vi "Read Data Type Information.vi"(8 "error in (no error)":errorcluster, 10 "Name":string, 11 "TwinCAT ADS in":refnum<class "TwinCAT ADS.lvclass">) -> (0 "error out":errorcluster, 1 "Data Type Information":T1 {"Category" items=["Unknown, None"=0, "Primitive"=1, "Alias"=2, "Enum"=3, "Array"=4, "Struct"=5, "FunctionBlock"=6, "Program"=7, "Function"=8, "SubRange"=9, "String"=10, "Bitset"=12, "Pointer"=13, "Union"=14, "Reference"=15, "Interface"=16]; "Type ID" items=["ADST_VOID"=0, "ADST_INT16"=2, "ADST_INT32"=3, "ADST_REAL32"=4, "ADST_REAL64"=5, "ADST_INT8"=16, "ADST_UINT8"=17, "ADST_UINT16"=18, "ADST_UINT32"=19, "ADST_INT64"=20, "ADST_UINT64"=21, "ADST_STRING"=30, "ADST_WSTRING"=31, "ADST_REAL80"=32, "ADST_BIT"=33, "ADST_MAXTYPES"=34, "ADST_BIGTYPE"=65]}, 3 "TwinCAT ADS out":refnum<class "TwinCAT ADS.lvclass">)   [LabVIEW 2018, in "TwinCAT ADS.lvclass"]
uses:
  TwinCAT ADS.lvclass
  Controls/Data Type Information.ctl
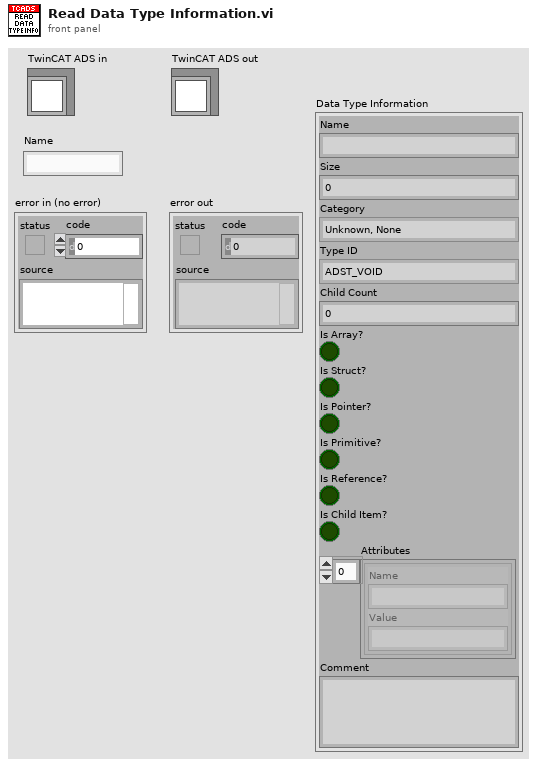
[diagram p1: front panel]
types:
  T1 = typedef "TwinCAT ADS.lvclass/Data Type Information.ctl" = cluster{"Name":string, "Size":i32, "Category":i32, "Type ID":i32, "Child Count":i32, "Is Array?":bool, "Is Struct?":bool, "Is Pointer?":bool, "Is Primitive?":bool, "Is Reference?":bool, "Is Child Item?":bool, "Attributes":cluster{"Name":string, "Value":string}[], "Comment":string}
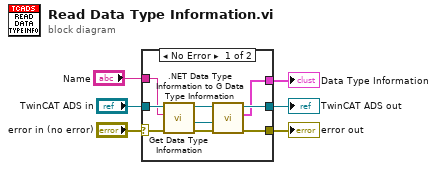
[diagram p0: block diagram]
diagram:
  n1 = case shown="No Error" "error in (no error)" {
    selector: "error in (no error)" -> [w11 w17]
    tunnel: [w10 w17] -> w5
    tunnel: [w9 w16] -> w3
    tunnel: "TwinCAT ADS in" -> [w15 w16]
    tunnel: "Name" -> [w8 _]
    tunnel: [w7 _] -> w1
    frame No Error {
      n2 = call-dynamic "Get Data Type Information.vi"("error in (no error)"=w11, "Name"=w8, "TwinCAT ADS in"=w15) -> ("error out"=w13:errorcluster, "Data Type Info"=w12:refnum<k24>, "TwinCAT ADS out"=w14:refnum<class "TwinCAT ADS.lvclass">)  [unwired: 6 in]
      n3 = call ".NET Data Type Information to G Data Type Information.vi"("error in (no error)"=w13, ".NET Data Type Information"=w12, "TwinCAT ADS in"=w14) -> ("error out"=w10:errorcluster, "Data Type Information"=w7:T1, "TwinCAT ADS out"=w9:refnum<class "TwinCAT ADS.lvclass">)  [unwired: 6 in]
    }
    frame Error {
    }
  }
  "error out" <- w5
  "TwinCAT ADS out" <- w3
  "Data Type Information" <- w1
